vi "Get CCD status.vi"(8 "error in (no error)":errorcluster, 11 "RxTx in":refnum<class "RxTx.lvclass">) -> (0 "error out":errorcluster, 3 "RxTx out":refnum<class "RxTx.lvclass">)   [LabVIEW 2018, in "RxTx.lvclass"]
uses:
  RxTx.lvclass
  RxTx.lvclass/RxTx.ctl
  Interface/Interface.lvclass
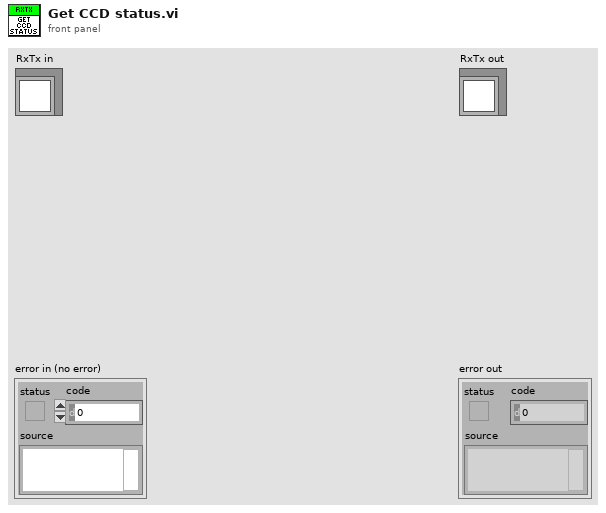
[diagram p1: front panel]
types:
  T1 = cluster{"CUBE_EXPOSURE_TIME":sgl, "CUBES_DONE":u16, "LAST_IMAGE_NAME":string, "DISK_SPACE":u16, "FRAMES_DONE":u16, "CCD_STATUS":string, "CURRENT_TEMPERATURE":i16, "TEMPERATURE_STATUS":string, "FRAME_EXPOSURE_TIME":u16, "CCD_ON_OFF":bool, "SERIAL_NUMBER":u16, "ACQUIRING":bool}
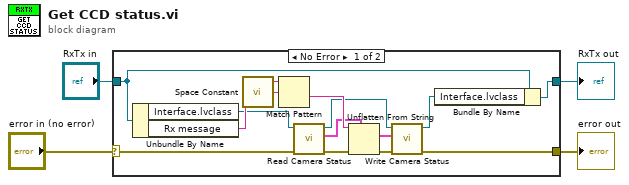
[diagram p0: block diagram]
diagram:
  n1 = case shown="No Error" "error in (no error)" {
    selector: "error in (no error)" -> [w9 w20]
    tunnel: [w14 w20] -> w3
    tunnel: [w12 w19] -> w1
    tunnel: "RxTx in" -> [w13 w19]
    frame No Error {
      n2 = Unbundle By Name(w13) -> ("Interface.lvclass"=w8:refnum<class "Interface.lvclass">, "Rx message"=w18:string)
      n3 = call <vilib>:"Space Constant.vi"() -> ("String"=w17:string)
      n4 = Match Pattern(string=w18, regular expression=w17) -> (after substring=w16:string)  [unwired: 1 in, 3 out]
      n5 = call "Read Camera Status.vi"("error in (no error)"=w9, "Interface in"=w8) -> ("error out"=w10:errorcluster, "Camera Status"=w5:T1, "Interface out"=w7:refnum<class "Interface.lvclass">)  [unwired: 7 in]
      n6 = Unflatten From String(type=w5, binary string=w16, error in (no error)=w10) -> (value=w6:T1, error out=w15:errorcluster)  [unwired: 2 in, 1 out]
      n7 = call "Write Camera Status.vi"("error in (no error)"=w15, "Camera Status"=w6, "Interface in"=w7) -> ("error out"=w14:errorcluster, "Interface out"=w11:refnum<class "Interface.lvclass">)  [unwired: 7 in]
      n8 = Bundle By Name(cluster=w13, "Interface.lvclass"=w11) -> (w12:refnum<class "RxTx.lvclass">)
    }
    frame Error {
    }
  }
  "error out" <- w3
  "RxTx out" <- w1
